vi "Help Message Bottom--constant.vi"() -> (3 "Help Message Bottom":string)   [LabVIEW 2025]
doc: "This constant contains the final part of the help message."
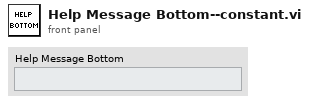
[diagram p1: front panel]
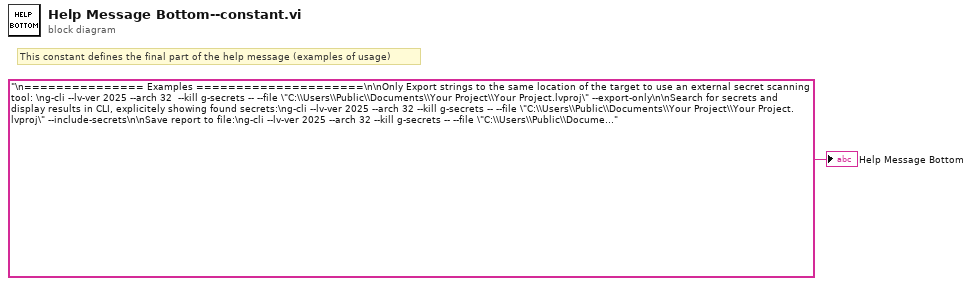
[diagram p0: block diagram]
diagram:
  # "This constant defines the final part of the help message (examples of usage)"
  "Help Message Bottom" <- "\n=============== Examples =====================\n\nOnly Export strings to the same location of the target to use an external secret scanning tool: \ng-cli --lv-ver 2025 --arch 32  --kill g-secrets -- --file \"C:\\Users\\Public\\Documents\\Your Project\\Your Project.lvproj\" --export-only\n\nSearch for secrets and display results in CLI, explicitely showing found secrets:\ng-cli --lv-ver 2025 --arch 32 --kill g-secrets -- --file \"C:\\Users\\Public\\Documents\\Your Project\\Your Project.lvproj\" --include-secrets\n\nSave report to file:\ng-cli --lv-ver 2025 --arch 32 --kill g-secrets -- --file \"C:\\Users\\Public\\Documents\\Your Project\\Your Project.lvproj\" --report \"C:\\Users\\Public\\Secrets.txt\"\n\n============================================"
